vi "Verify Blink LE.vi"(0 "GEA2 Reference In":refnum<k24>, 1 "Standalone":bool, 2 "Blinking LED":T1, 5 "Initial Timeout (s)":dbl, 7 "Retry Count":i32, 9 "Max Blink Rate (sec)":dbl, 11 "Error In":errorcluster, 12 "Ignore Brightness":bool) -> (4 "GEA2 Reference Out":refnum<k24>, 6 "Pass/Fail?":bool, 8 "Report Text":string, 10 "Blink Times (s)":dbl[](array[numeric]), 14 "Binary Number Out":u32, 15 "Error Out":errorcluster)   [LabVIEW 2016, in "Centauro.lvlib"]
doc: "This VI is used to verify that a particular LED is blinking on the LEUI."
uses:
  Projects/Centauro.lvlib
  Q:/Common/DLLs/GEA3/GeaCommunication.dll
  Common/DLLs/GEA3/GeaCommunication.dll
  Common/LabVIEW GEA2 Toolkit/LabVIEW_GEA2_Toolkit.lvlibp/type defs/Source_Destination.ctl
  Common/LabVIEW GEA2 Toolkit/LabVIEW_GEA2_Toolkit.lvlibp
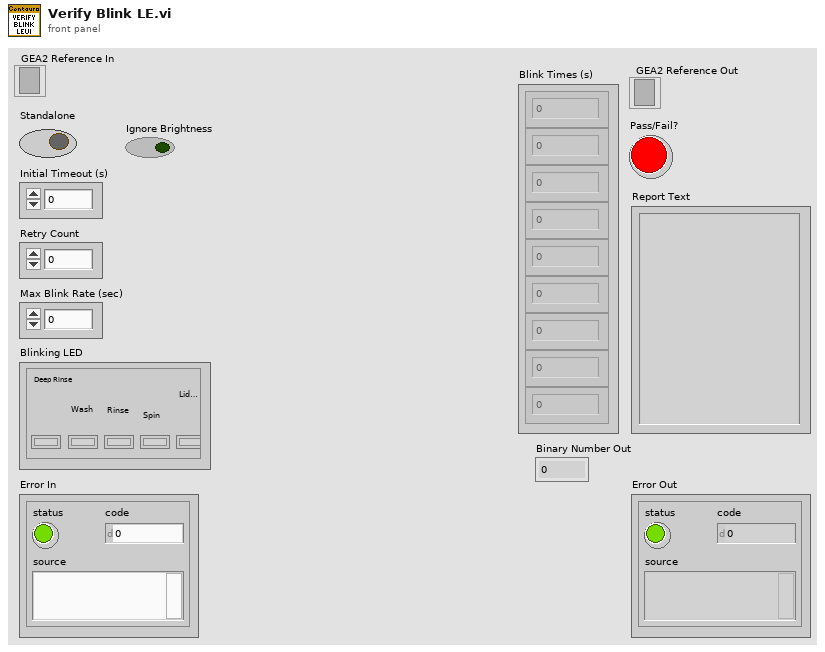
[diagram p1: front panel]
types:
  T1 = cluster{"Deep Rinse":bool, "Wash":bool, "Rinse":bool, "Spin":bool, "Lid Lock":bool}
  T2 = typedef "LabVIEW_GEA2_Toolkit.lvlibp/Source_Destination.ctl" = cluster{"Source":u8, "Destination":u8}
  T3 = typedef "LED Status OOB.ctl" = enum32{"Off", "On", "Blink"}
  T4 = cluster{"Deep Rinse":T3, "Wash":T3, "Rinse":T3, "Spin":T3, "Lid Lock":T3}
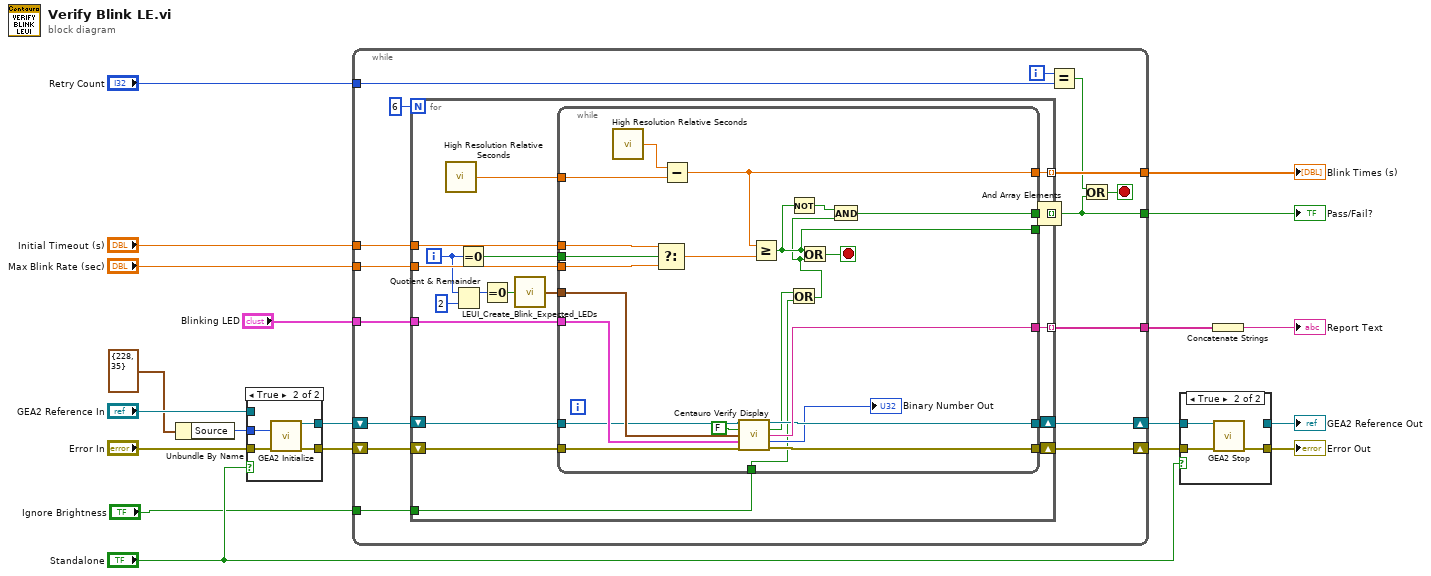
[diagram p0: block diagram]
diagram:
  n1 = Unbundle By Name(T2 {"Source"=228, "Destination"=35} ("GEA Inputs")) -> ("Source"=w19:u8)
  n2 = case shown="True" "Standalone" {
    tunnel: "Error In" -> [w22 w26]
    tunnel: w19 -> [_ w25]
    tunnel: [w21 w24] -> w11
    tunnel: [w22 w23] -> w10
    tunnel: "GEA2 Reference In" -> [w21 _]
    frame False {
    }
    frame True {
      n3 = call "GEA2 Initialize.vi"("Source Address"=w25, "error in"=w26) -> ("GEA2 Reference Out"=w24:refnum<k24>, "error out"=w23:errorcluster)  [unwired: 11 in, 1 out]
    }
  }
  n4 = while {
    tunnel: "Max Blink Rate (sec)" -> [w43]
    tunnel: [w32] -> w5
    tunnel: [w42] -> w12
    tunnel: "Blinking LED" -> [w37]
    tunnel: "Initial Timeout (s)" -> [w36]
    shift-right: [w39] -> w9
    shift-left: w11 -> [w41]
    shift-right: [w38] -> w8
    shift-left: w10 -> [w40]
    tunnel: [w35] -> w6
    tunnel: "Retry Count" -> [w29]
    tunnel: "Ignore Brightness" -> [w27]
    i -> [w30]
    stop <- w31 stop-if-true
    n5 = for {
      N: 6 -> [_]
      shift-right: [w60] -> w38
      shift-left: w40 -> [w61]
      shift-right: [w59] -> w39
      shift-left: w41 -> [w58]
      tunnel: w43 -> [w56]
      tunnel: [w54] -> w34 mode=indexing
      tunnel: [w51] -> w35 mode=indexing
      tunnel: [w55] -> w42 mode=indexing
      tunnel: w37 -> [w50]
      tunnel: w36 -> [w52]
      tunnel: w27 -> [w44]
      i -> [w45]
      n6 = call <vilib>:"High Resolution Relative Seconds.vi"() -> ("relative seconds"=w57:dbl)
      n7 = Quotient & Remainder(x=w45, y=2) -> (x-y*floor(x/y)=w48:i32)  [unwired: 1 out]
      n8 = Equal To 0?(x=w45) -> (x = 0?=w53:bool)
      n9 = Equal To 0?(x=w48) -> (x = 0?=w47:bool)
      n10 = call "LEUI_Create_Blink_Expected_LEDs.vi"("Boolean"=w47) -> ("Expect LED's Out"=w46:T4)  [unwired: 14 in]
      n11 = while {
        tunnel: w61 -> [w67]
        tunnel: [w70] -> w60
        tunnel: [w71] -> w59
        tunnel: w58 -> [w66]
        tunnel: w57 -> [w83]
        tunnel: w56 -> [w78]
        tunnel: [w81] -> w54
        tunnel: [w82] -> w55
        tunnel: w53 -> [w75]
        tunnel: w50 -> [w68]
        tunnel: w52 -> [w79]
        tunnel: [w72] -> w51
        tunnel: w46 -> [w69]
        tunnel: [w74] -> _
        tunnel: w44 -> [w62]
        stop <- w80 stop-if-true
        n12 = call <vilib>:"High Resolution Relative Seconds.vi"() -> ("relative seconds"=w84:dbl)
        n13 = Select(t=w79, s=w75, f=w78) -> (s? t:f=w77:dbl)
        n14 = Subtract(x=w84, y=w83) -> (x-y=w82:dbl)
        n15 = call "Centauro Verify Display.vi"("GEA2 Reference In"=w66, "Standalone?"=FALSE, "Expected LED Status"=w69, "Care"=w68, "Error In"=w67) -> ("GEA2 Reference Out"=w71:refnum<k24>, "Pass/Fail?"=w65:bool, "Report Text"=w72:string, "Binary Number Out"=→"Binary Number Out":u32, "Error Out"=w70:errorcluster)  [unwired: 6 in]
        n16 = Greater Or Equal?(x=w82, y=w77) -> (x >= y?=w74:bool)
        n17 = Not(x=w74) -> (.not. x?=w76:bool)
        n18 = Or(x=w65, y=w62) -> (x .or. y?=w64:bool)
        n19 = Or(x=w74, y=w64) -> (x .or. y?=w80:bool)
        n20 = And(x=w76, y=w64) -> (x .and. y?=w81:bool)
      }
    }
    n21 = And Array Elements(Boolean array=w34) -> (logical AND=w32:bool)
    n22 = Equal?(x=w30, y=w29) -> (x = y?=w33:bool)
    n23 = Or(x=w33, y=w32) -> (x .or. y?=w31:bool)
  }
  "Pass/Fail?" <- w5
  "Blink Times (s)" <- w12
  n24 = case shown="True" "Standalone" {
    tunnel: w8 -> [w86 w89]
    tunnel: [w86 w88] -> w17
    tunnel: w9 -> [w85 w87]
    tunnel: [w85 _] -> w15
    frame False {
    }
    frame True {
      n25 = call "GEA2 Stop.vi"("GEA2 Reference In"=w87, "Error In"=w89) -> ("Error Out"=w88:errorcluster)  [unwired: 13 in]
    }
  }
  "GEA2 Reference Out" <- w15
  "Error Out" <- w17
  n26 = Concatenate Strings(w6) -> (→"Report Text":string)
